vi "BodyTextCoordinates.vi"(9 "Body Text":T2={"Line 1 text"="", "Line 2 text"="", "Line 3 text"="", "Line 4 text"="", "Line 1 color"=0, "Line 2 color"=0, "Line 3 color"=0, "Line 4 color"=0, "Body Text Spec"={"Font"="", "Alignment"=0, "Size"=3}, "Center text vertically"=FALSE, "Capitalize Text"=FALSE} {"Body Text Spec"."Alignment" items=["left", "center", "right"]}, 10 "Path and Icon Template":T1, 11 "Icon.lvclass in":refnum<class "Icon.lvclass">) -> (1 "Coordinates":cluster{"x":i16, "y":i16}[](array[cluster]), 2 "color out":u32[](array[numeric]), 3 "Lines out":string[](array[string]))   [LabVIEW 2020, in "Icon Framework.lvclass"]
doc: "Determines the position of each line of the body text."
uses:
  <vilib>/LabVIEW Icon API/lv_icon/Classes/Icon Framework/Icon Framework.lvclass
  <vilib>/LabVIEW Icon API/lv_icon/Controls/BodyText.ctl
  <vilib>/LabVIEW Icon API/lv_icon/Controls/Font.ctl
  <vilib>/LabVIEW Icon API/lv_icon/Controls/Alignment.ctl
  <vilib>/LabVIEW Icon API/lv_icon/Classes/Icon/Icon.lvclass
  <vilib>/LabVIEW Icon API/lv_icon/Controls/Graphic.ctl
  <vilib>/LabVIEW Icon API/lv_icon/Controls/BodyTextPosition.ctl
  <vilib>/LabVIEW Icon API/lv_icon/lv_icon.lvlib
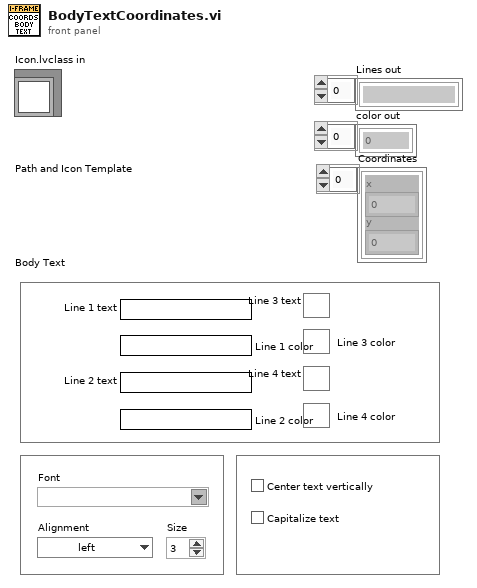
[diagram p1: front panel]
types:
  T1 = typedef "Graphic.ctl" = cluster{"Rectangle":cluster{"left":i16, "top":i16, "right":i16, "bottom":i16}, "Path":path, "Image":picture, "Filter":string, "FileName":string}
  T2 = typedef "BodyText.ctl" = cluster{"Line 1 text":string, "Line 2 text":string, "Line 3 text":string, "Line 4 text":string, "Line 1 color":u32, "Line 2 color":u32, "Line 3 color":u32, "Line 4 color":u32, "Body Text Spec":cluster{"Font":T3, "Alignment":T4, "Size":u8}, "Center text vertically":bool, "Capitalize Text":bool}
  T3 = typedef "Font.ctl" = string
  T4 = typedef "Alignment.ctl" = u16
  T5 = typedef "IEColor.ctl" = u32
  T6 = typedef "BodyTextPosition.ctl" = enum8{"Default", "All lines centered"}
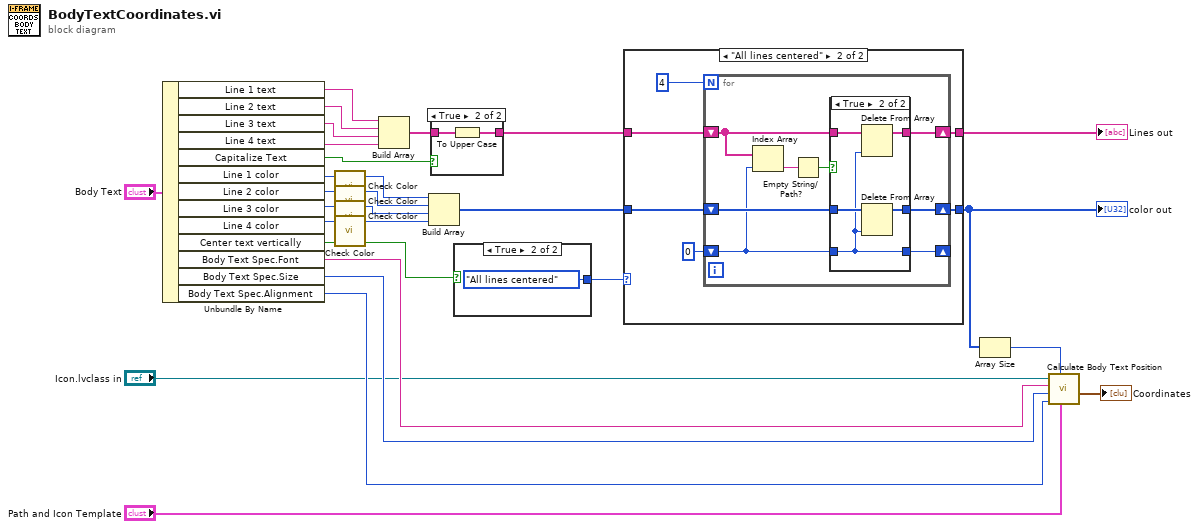
[diagram p0: block diagram]
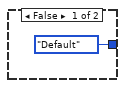
[diagram p3: hidden frame]
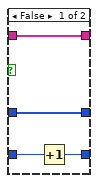
[diagram p5: hidden frame]
diagram:
  n1 = Unbundle By Name("Body Text") -> ("Line 1 text"=w20:string, "Line 2 text"=w21:string, "Line 3 text"=w22:string, "Line 4 text"=w23:string, "Capitalize Text"=w18:bool, "Line 1 color"=w14:u32, "Line 2 color"=w15:u32, "Line 3 color"=w16:u32, "Line 4 color"=w17:u32, "Center text vertically"=w9:bool, "Body Text Spec.Font"=w5:T3, "Body Text Spec.Size"=w4:u8, "Body Text Spec.Alignment"=w3:T4)
  n2 = call <vilib>:"Check Color.vi"("Color in"=w14) -> ("Color out"=w10:T5)  [unwired: 26 out]
  n3 = call <vilib>:"Check Color.vi"("Color in"=w15) -> ("Color out"=w11:T5)  [unwired: 26 out]
  n4 = call <vilib>:"Check Color.vi"("Color in"=w16) -> ("Color out"=w12:T5)  [unwired: 26 out]
  n5 = call <vilib>:"Check Color.vi"("Color in"=w17) -> ("Color out"=w13:T5)  [unwired: 26 out]
  n6 = Build Array(w20, w21, w22, w23) -> (w19:string[])
  n7 = Build Array(w10, w11, w12, w13) -> (w7:T5[])
  n8 = case shown="True" w18 {
    tunnel: w19 -> [w29 w31]
    tunnel: [w29 w30] -> w8
    frame False {
    }
    frame True {
      n9 = To Upper Case(1:w31) -> (0:w30:string[])
    }
  }
  n10 = case shown="True" w9 {
    tunnel: [BodyTextPosition."Default" ("AC Text?") BodyTextPosition."All lines centered" ("AC Text?")] -> w6
    frame False {
    }
    frame True {
    }
  }
  n11 = case shown="\"All lines centered\"" w6 {
    tunnel: [w35 w41] -> w28
    tunnel: [w34 w40] -> w27
    tunnel: w7 -> [w34 w38]
    tunnel: w8 -> [w35 w37]
    frame "Default", Default {
    }
    frame "All lines centered" {
      n12 = for {
        N: 4 -> [_]
        shift-right: [w46] -> w41
        shift-left: w37 -> [w47]
        shift-right: [w45] -> w40
        shift-left: w38 -> [w44]
        shift-right: [w42] -> _
        shift-left: i16 0 -> [w43]
        n13 = Index Array(array=w47, index=w43) -> (element=w49:string)
        n14 = Empty String/Path?(string/path=w49) -> (empty?=w48:bool)
        n15 = case shown="True" w48 {
          tunnel: w47 -> [w53 w58]
          tunnel: [w53 w57] -> w46
          tunnel: [w52 w55] -> w45
          tunnel: w44 -> [w52 w56]
          tunnel: w43 -> [w51 w54]
          tunnel: [w50 w54] -> w42
          frame False {
            n16 = Increment(x=w51) -> (x+1=w50:i16)
          }
          frame True {
            n17 = Delete From Array(array=w58, index=w54) -> (array with subset deleted=w57:string[])  [unwired: 1 in, 1 out]
            n18 = Delete From Array(array=w56, index=w54) -> (array with subset deleted=w55:T5[])  [unwired: 1 in, 1 out]
          }
        }
      }
    }
  }
  "Lines out" <- w28
  "color out" <- w27
  n19 = Array Size(array=w27) -> (size(s)=w25:i32)
  n20 = call <vilib>:"Calculate Body Text Position.vi"("Path & Icon"="Path and Icon Template", "# lines"=w25, "horizontal"=w3, "Size"=w4, "Font Name:"=w5, "Icon.lvclass in"="Icon.lvclass in") -> ("Locations"=→"Coordinates":cluster{i16, i16}[])  [unwired: 1 in, 4 out]
